vi "SMO.TimedLoop.GenerateNewValueEvent.vi"(8 "error in (no error)":errorcluster, 10 "New Value":dbl, 11 "SMO.TimedLoop":refnum<class "SMO.TimedLoop.lvclass">) -> (0 "error out":errorcluster, 3 "SMO.TimedLoop out":refnum<class "SMO.TimedLoop.lvclass">)   [LabVIEW 2019, in "SMO.TimedLoop.lvclass"]
doc: "---------------------------------------------------------------\nJKI State Machine Objects™\nhttp://jki.net/state-machine-objects/\nCopyright (C) 2005-2015, JKI <info@jki.net>\nALL RIGHTS RESERVEDJKI State Machine Objects (SMO) 1.0.0.5\nJKI - JKI\nCopyright (c) 2016, JKI"
uses:
  SMO.TimedLoop.lvclass
panel:
  # "For instructions on how to use the JKI State Machine Objects, examples and video tutorials, visit:\nhttp://jki.net/state-machine-objects/\n\nJKI State Machine Objects™\nhttp://jki.net/state-machine-objects/\nCopyright (C) 2005-2015, JKI <info@jki.net>\nALL RIGHTS RESERVED"
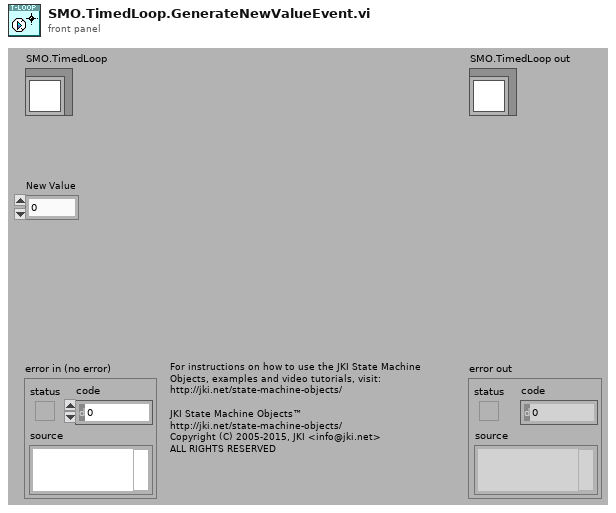
[diagram p1: front panel]
types:
  T1 = typedef "SMO.TimedLoop.lvclass/PublicEvents--Cluster.ctl" = cluster{"Setpoint Changed":refnum<user-event>, "Value Changed":refnum<user-event>}
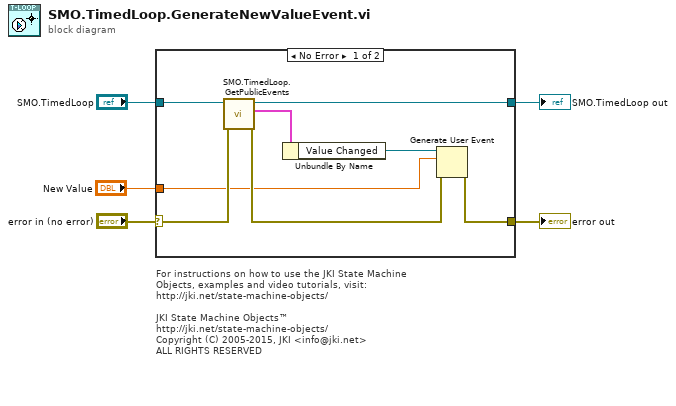
[diagram p0: block diagram]
diagram:
  # "For instructions on how to use the JKI State Machine Objects, examples and video tutorials, visit:\nhttp://jki.net/state-machine-objects/\n\nJKI State Machine Objects™\nhttp://jki.net/state-machine-objects/\nCopyright (C) 2005-2015, JKI <info@jki.net>\nALL RIGHTS RESERVED"
  n1 = case shown="No Error" "error in (no error)" {
    selector: "error in (no error)" -> [w10 w14]
    tunnel: "SMO.TimedLoop" -> [w11 w15]
    tunnel: [w13 w14] -> w4
    tunnel: [w12 w15] -> w3
    tunnel: "New Value" -> [w6 _]
    frame No Error {
      n2 = call "SMO.TimedLoop.GetPublicEvents.vi"("error in (no error)"=w10, "SMO.TimedLoop"=w11) -> ("error out"=w8:errorcluster, "my Public Events"=w7:T1, "SMO.TimedLoop out"=w12:refnum<class "SMO.TimedLoop.lvclass">)  [unwired: 7 in]
      n3 = Unbundle By Name(w7) -> ("Value Changed"=w9:refnum<user-event>)
      n4 = Generate User Event(user event=w9, event data cluster=w6, error in=w8) -> (error out=w13:errorcluster)  [unwired: 1 in, 1 out]
    }
    frame Error {
    }
  }
  "error out" <- w4
  "SMO.TimedLoop out" <- w3
